vi "Weather Station UI.vi"() -> ()   [LabVIEW 2025]
doc: "This is the main VI in the Weather Station project. It contains the user interface for a temperature warning system. Temperature is retrieved every half second; data is logged when a warning has occurred."
uses:
  Weather Station States.ctl
  Supporting Files/Weather Data.ctl
  Instance           2 26Saved   Weather Station UI .vi
panel:
  in  "Always log":bool
  out "Warning":string
  in  "Lower Limit":dbl=20.0
  in  "Upper Limit":dbl=30.0
  in  "Stop Button":bool
  out "Temperature History":dbl(graph)
  # "Temperature Ranges (C)"
  # "Freeze"
  # "Heat \nStroke"
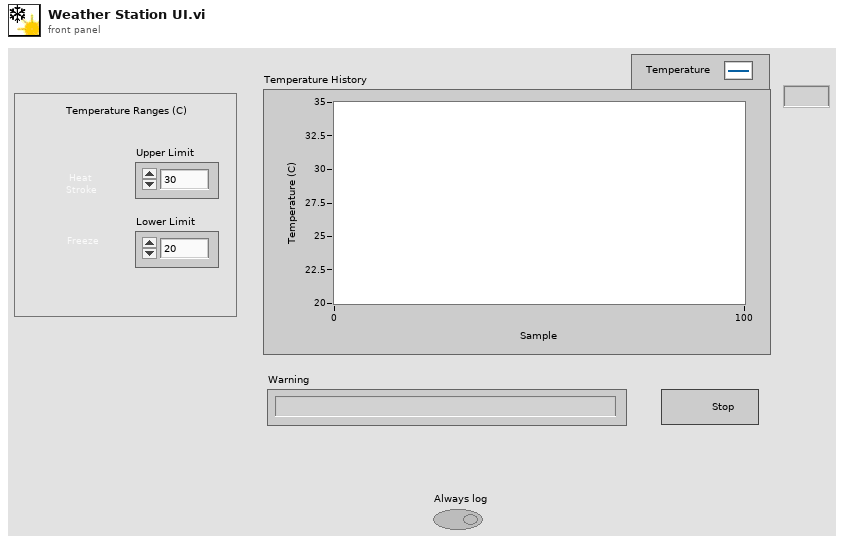
[diagram p1: front panel]
types:
  T1 = typedef "Weather Data.ctl" = cluster{"Current Temperature":dbl, "Max Temperature":dbl, "Min Temperature":dbl, "Temperature Warning?":bool, "Temperature Warning Text":string}
  T2 = typedef "Weather Station States.ctl" = enum16{"Acquisition", "Analysis", "Datal Log", "Time Check"}
  T3 = enum16{"open", "replace", "create", "open or create", "replace or create", "replace or create with confirmation"}
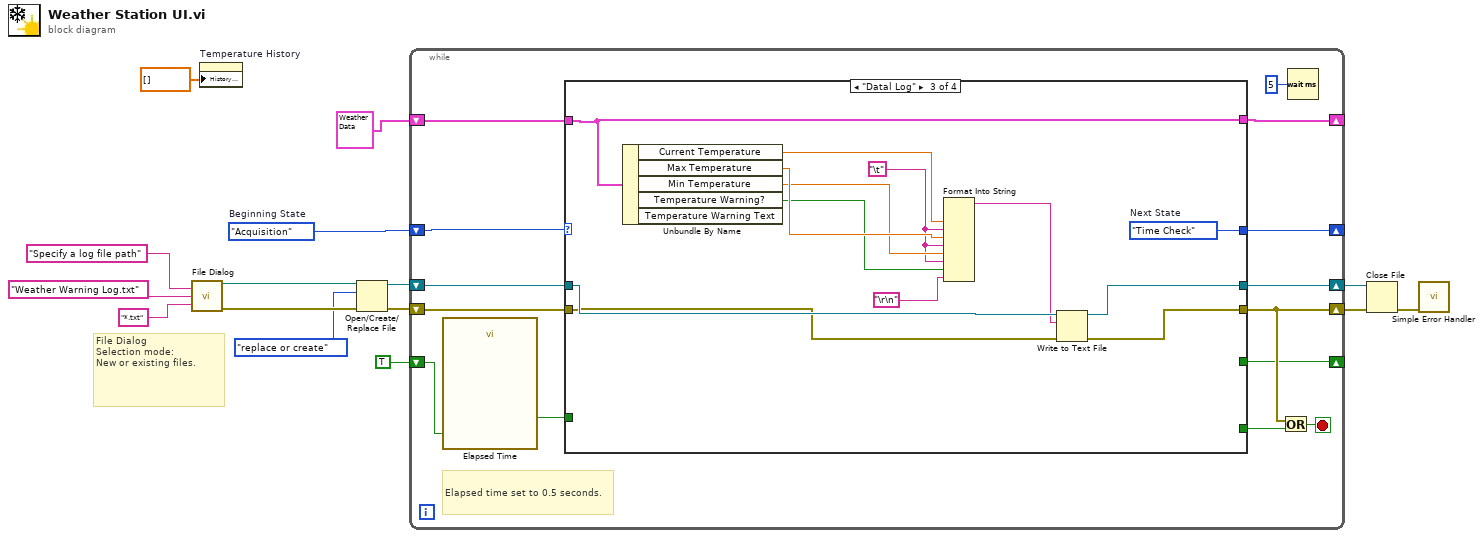
[diagram p0: block diagram]
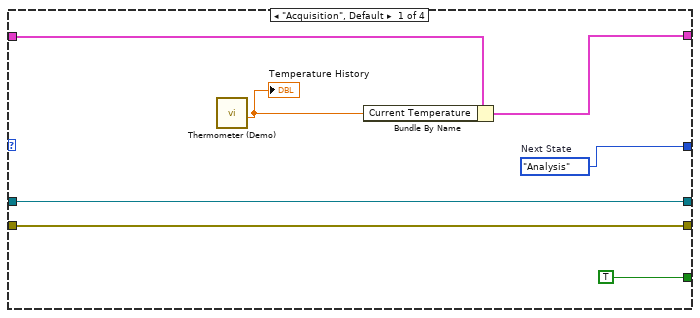
[diagram p2: hidden frame]
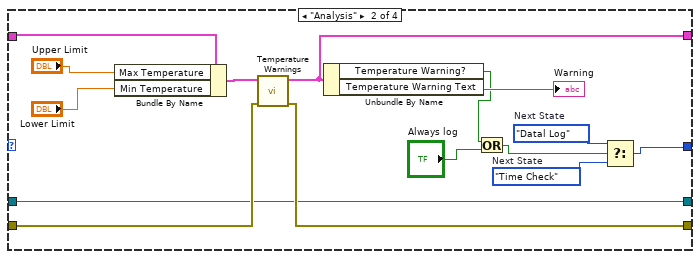
[diagram p3: hidden frame]
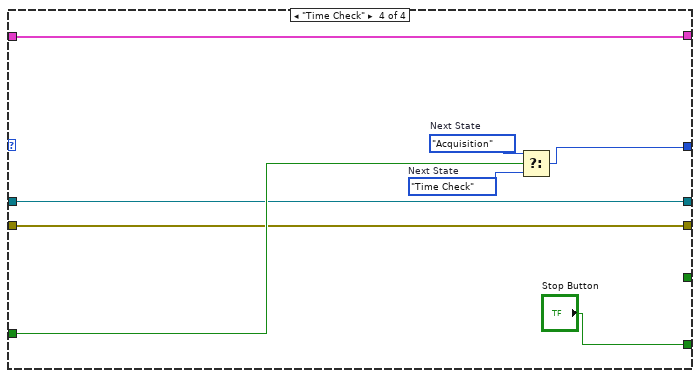
[diagram p4: hidden frame]
diagram:
  w3 = Weather_Station_States."Acquisition"  # Beginning State
  # "File Dialog\nSelection mode:\nNew or existing files."
  n1 = call "File Dialog"("prompt"="Specify a log file path", "default name"="Weather Warning Log.txt", "pattern (all files)"="*.txt" ("pattern label")) -> ("selected path"=w9:path, "error out"=w6:errorcluster)  [unwired: 9 in, 2 out]
  n2 = property on="Temperature History" class="WFChart (strict)"("History Data"=dbl[] []) -> ()  [unwired: 2 in, 2 out]
  n3 = Open/Create/Replace File(file path (use dialog)=w9, error in=w6, operation (0:open)=T3."replace or create") -> (refnum out=w11:refnum<file>, error out=w10:errorcluster)  [unwired: 3 in, 1 out]
  n4 = while {
    shift-right: [w22] -> w15
    shift-left: w10 -> [w29]
    shift-right: [w27] -> w14
    shift-left: w11 -> [w26]
    shift-right: [w17] -> _
    shift-left: TRUE ("stop") -> [w24]
    shift-right: [w18] -> _
    shift-left: w3 -> [w21]
    shift-right: [w19] -> _
    shift-left: T1 {"Current Temperature"=0.0, "Max Temperature"=0.0, "Min Temperature"=0.0, "Temperature Warning?"=FALSE, "Temperature Warning Text"="No Warning"} ("Weather Data In") -> [w20]
    stop <- w28 stop-if-true
    # "Elapsed time set to 0.5 seconds."
    n5 = call "Elapsed Time"("Reset"=w24) -> ("Time has Elapsed"=w23:bool)  [unwired: 11 in, 7 out]
    n6 = case shown="\"Datal Log\"" w21 {
      tunnel: [w35 w47 w53 w66] -> w22
      tunnel: w29 -> [w35 w48 w54 w66]
      tunnel: [w36 w43 w52 w69] -> w27
      tunnel: w26 -> [w36 w43 w56 w69]
      tunnel: w23 -> [_ _ _ w70]
      tunnel: w20 -> [w33 w41 w64 w67]
      tunnel: [w32 w40 w64 w67] -> w19
      tunnel: [w31 w44 w63 w68] -> w18
      tunnel: [TRUE ("stop") _ _ _] -> w17
      tunnel: [_ _ _ "Stop Button"] -> w16
      frame "Acquisition", Default {
        w31 = Weather_Station_States."Analysis"  # Next State
        n7 = call "Thermometer (Demo).vi"() -> ("Temperature Value"=w34:dbl)  [unwired: 11 in]
        "Temperature History" <- w34
        n8 = Bundle By Name(cluster=w33, "Current Temperature"=w34) -> (w32:T1)
      }
      frame "Analysis" {
        w42 = Weather_Station_States."Time Check"  # Next State
        w45 = Weather_Station_States."Datal Log"  # Next State
        n9 = Bundle By Name(cluster=w41, "Max Temperature"="Upper Limit", "Min Temperature"="Lower Limit") -> (w49:T1)
        n10 = call "Temperature Warnings.vi"("Error In"=w48, "Weather Data In"=w49) -> ("Error Out"=w47:errorcluster, "Weather Data Out"=w40:T1)  [unwired: 8 in]
        n11 = Unbundle By Name(w40) -> ("Temperature Warning?"=w38:bool, "Temperature Warning Text"=→"Warning":string)
        n12 = Or(x=w38, y="Always log") -> (x .or. y?=w39:bool)
        n13 = Select(t=w45, s=w39, f=w42) -> (s? t:f=w44:T2)
      }
      frame "Datal Log" {
        w59 = "\t"
        w63 = Weather_Station_States."Time Check"  # Next State
        n14 = Unbundle By Name(w64) -> ("Current Temperature"=w62:dbl, "Max Temperature"=w61:dbl, "Min Temperature"=w60:dbl, "Temperature Warning?"=w58:bool)  [unwired: 1 out]
        n15 = Format Into String(w62, w59, w61, w59, w60, w59, w58, "\r\n") -> (resulting string=w55:string)  [unwired: 3 in, 1 out]
        n16 = Write to Text File(file (use dialog)=w56, text=w55, error in=w54) -> (refnum out=w52:refnum<file>, error out=w53:errorcluster)  [unwired: 1 in, 1 out]
      }
      frame "Time Check" {
        w71 = Weather_Station_States."Time Check"  # Next State
        w72 = Weather_Station_States."Acquisition"  # Next State
        n17 = Select(t=w72, s=w70, f=w71) -> (s? t:f=w68:T2)
      }
    }
    n18 = Or(x=w22, y=w16) -> (x .or. y?=w28:bool)
    n19 = Wait (ms)(milliseconds to wait=u32 5 ("y")) -> ()  [unwired: 1 out]
  }
  n20 = Close File(refnum=w14, error in=w15) -> (error out=w13:errorcluster)  [unwired: 1 out]
  n21 = call <vilib>:"Simple Error Handler.vi"("error in (no error)"=w13) -> ()  [unwired: 4 in, 5 out]
